vi "MGCC_MdlMgmt_Graphic.vi"() -> ()   [LabVIEW 2016]
doc: "-----------------------------------------------------------------------------------------------------------------------\nCopyright <2019> <The University of Tennessee at Knoxville and the University of Tennessee Research Foundation>\nThis software is released under BSD-3 \nhttps://opensource.org/licenses/BSD-3-Clause \nAdditional license options available at https://utrf.tennessee.edu/industry/sample-agreements/\n-----------------------------------------------------------------------------------------------------------------------\n\nThis VI is designed to initize the SHE215 model with graphic (2D double array).-----------------------------"
uses:
  <vilib>/imath/engines/lvmath2/RunTimeEngine/NodeEndStatement/NIMS_NodeEndStatement_Output.vi
  <instcachedir>/0/NIMS_NodeEndStatement_Output_53EC0D466D134D7ABD903AC30B43404B.lvgen/NIMS_NodeEndStatement_Output_53EC0D466D134D7ABD903AC30B43404B_010.vi
  <vilib>/imath/engines/lvmath2/RunTimeEngine/ErrorHandling/NIMS_Finalize Error.vi
panel:
  out "array":dbl[][](array[numeric])
  out "text":string
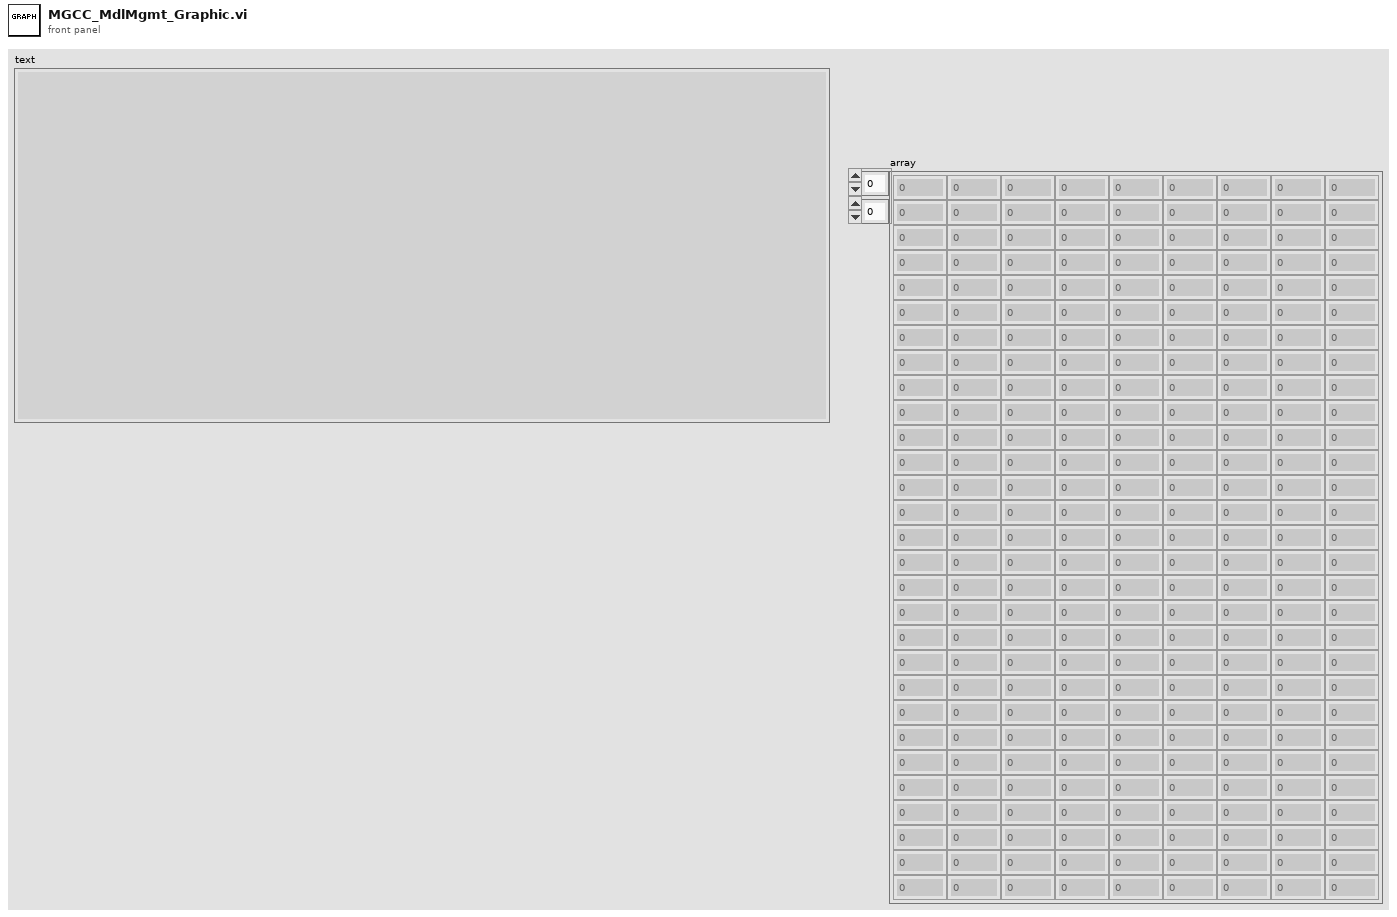
[diagram p1: front panel]
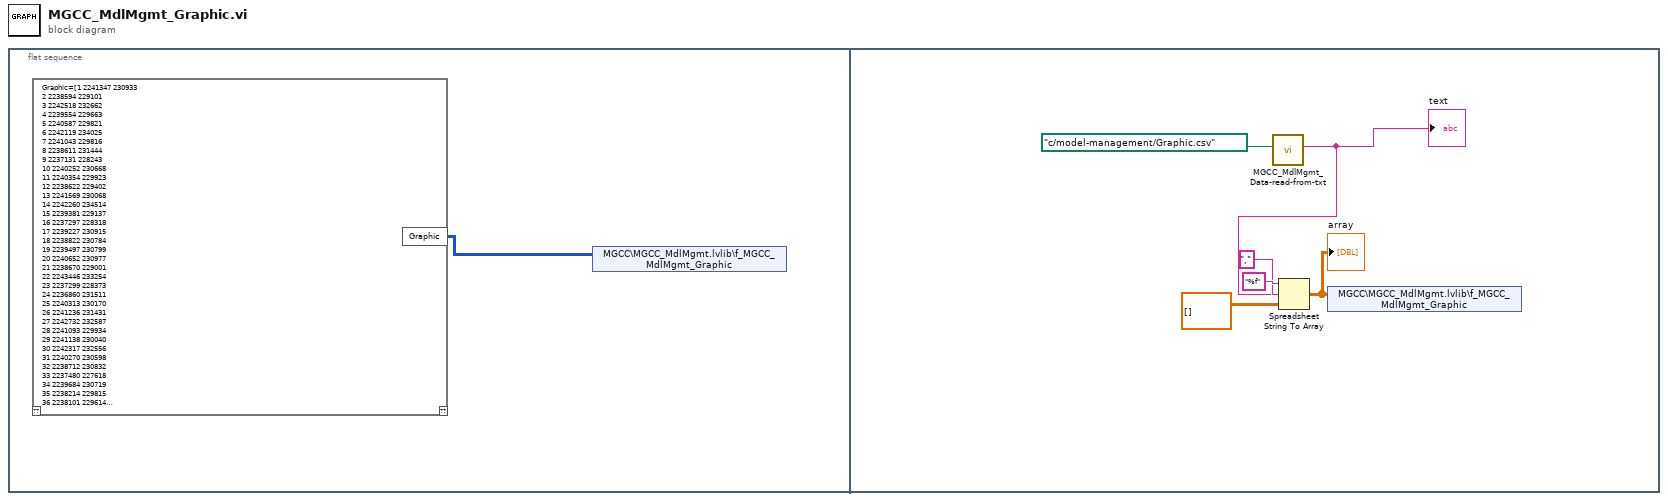
[diagram p0: block diagram]
diagram:
  n1 = flat-sequence {
    frame #0 {
      n2 = mathscript code="Graphic=[1\t2241347\t230933\n2\t2238594\t229101\n3\t2242518\t232662\n4\t2239554\t229663\n5\t2240587\t229821\n6\t2242119\t234025\n7\t2241043\t229816\n8\t2238611\t231444\n9\t2237131\t228243\n10\t2240252\t230668\n11\t2240354\t229923\n12\t2238622\t229402\n13\t2241569\t230068\n14\t2242260\t234514\n15\t2239381\t229137\n16\t2237297\t228318\n17\t2239227\t230915\n18\t2238822\t230784\n19\t2239497\t230799\n20\t2240652\t230977\n21\t2238670\t229001\n22\t2243446\t233254\n23\t2237299\t228373\n24\t2236860\t231511\n25\t2240313\t230170\n26\t2241236\t231431\n27\t2242732\t232587\n28\t2241093\t229934\n29\t2241138\t230040\n30\t2242317\t232556\n31\t2240270\t230598\n32\t2238712\t230832\n33\t2237480\t227618\n34\t2239684\t230719\n35\t2238214\t229815\n36\t2238101\t229614\n37\t2239201\t229854\n38\t2239291\t230583\n39\t2239052\t228410\n40\t2237867\t229724\n41\t2238322\t229509\n42\t2238145\t229033\n43\t2241409\t230629\n44\t2239661\t229599\n45\t2242631\t234355\n46\t2238950\t231034\n47\t2237485\t228516\n48\t2243165\t233311\n49\t2239827\t230147\n50\t2238730\t230867\n51\t2239618\t228552\n52\t2240805\t229721\n53\t2237071\t228122\n54\t2240553\t230476\n55\t2242445\t234436\n56\t2239862\t230630\n57\t2242511\t233856\n58\t2238251\t229036\n59\t2237800\t227534\n60\t2243409\t233119\n61\t2240015\t230483\n62\t2236935\t228092\n63\t2237312\t232477\n64\t2237562\t228888\n65\t2240884\t230680\n66\t2238941\t232437\n67\t2243265\t234127\n68\t2238371\t230913\n69\t2239407\t230840\n70\t2240819\t231106\n71\t2239293\t228944\n72\t2240694\t229147\n73\t2238608\t230876\n74\t2239967\t230467\n75\t2239254\t228857\n76\t2239884\t230123\n77\t2238139\t227705\n78\t2238429\t229814\n79\t2237539\t229577\n80\t2241020\t230274\n81\t2240648\t229500\n82\t2238544\t231292\n83\t2237163\t231970\n84\t2240407\t230787\n85\t2243126\t234150\n86\t2236331\t230503\n87\t2240695\t230810\n88\t2238013\t227700\n89\t2237806\t228632\n90\t2238369\t229205\n91\t2237392\t229065\n92\t2241605\t232088\n93\t2240971\t230678\n94\t2238496\t229227\n95\t2242252\t233968\n96\t2241024\t229627\n97\t2237160\t228190\n98\t2239057\t230683\n99\t2241692\t231790\n100\t2238315\t229898\n101\t2241513\t230126\n102\t2240441\t230483\n103\t2242556\t232451\n104\t2238193\t229569\n105\t2237909\t228485\n106\t2237588\t229745\n107\t2240416\t230399\n108\t2238691\t229455\n109\t2239672\t230218\n110\t2236545\t230430\n111\t2238502\t231201\n112\t2241109\t229619\n113\t2237475\t228378\n114\t2238404\t230985\n115\t2239460\t229314\n116\t2237463\t229313\n117\t2240662\t230430\n118\t2236585\t227775\n119\t2241301\t231156\n120\t2237758\t228734\n121\t2239041\t230995\n122\t2236537\t230356\n123\t2236982\t227856\n124\t2239904\t230328\n125\t2237593\t229764\n126\t2238822\t231087\n127\t2243437\t233385\n128\t2240694\t230934\n129\t2238929\t231349\n130\t2241383\t230757\n131\t2240228\t229979\n132\t2239104\t228525\n133\t2243389\t233847\n134\t2236970\t228044\n135\t2240458\t229249\n136\t2237802\t227555\n137\t2238822\t229476\n138\t2237406\t228378\n139\t2241100\t229599\n140\t2239788\t228942\n141\t2242888\t234252\n142\t2240379\t230317\n143\t2237539\t228300\n144\t2239271\t229185\n145\t2236506\t230371\n146\t2236757\t227878\n147\t2238506\t229643\n148\t2240011\t230580\n149\t2240999\t229712\n150\t2243272\t234087\n151\t2237850\t227910\n152\t2237128\t231945\n153\t2242901\t232717\n154\t2236312\t230462\n155\t2240039\t229436\n156\t2237498\t229438\n157\t2241100\t231247\n158\t2240856\t230345\n159\t2239673\t228677\n160\t2238499\t229306\n161\t2239171\t228674\n162\t2241801\t231876\n163\t2241419\t230644\n164\t2237651\t228167\n165\t2241934\t232688\n166\t2239653\t229002\n167\t2241022\t231263\n168\t2241891\t234123\n169\t2243556\t233778\n170\t2237387\t228440\n171\t2236902\t227959\n172\t2236849\t231114\n173\t2238907\t232116\n174\t2239695\t229844\n175\t2238768\t229516\n176\t2236864\t227960\n177\t2242040\t232053\n178\t2237639\t229831\n179\t2240087\t230455\n180\t2241449\t230437\n181\t2240583\t229195\n182\t2242723\t233763\n183\t2240756\t230390\n184\t2240736\t230166\n185\t2242528\t234106\n186\t2243117\t232884\n187\t2243400\t233101\n188\t2239885\t229503\n189\t2243413\t234038\n190\t2240702\t230089\n191\t2236702\t227897\n192\t2239726\t228800\n193\t2239178\t229884\n194\t2238296\t229149\n195\t2239531\t229475\n196\t2239198\t229219\n197\t2239865\t230367\n198\t2237976\t227619\n199\t2240693\t229602\n200\t2236666\t230842\n201\t2238390\t229145\n202\t2240924\t229671\n203\t2237641\t227582\n204\t2237660\t228651\n205\t2238243\t228980\n206\t2238114\t229733\n207\t2242322\t232271\n208\t2240781\t230727\n209\t2243537\t233574\n210\t2240334\t229309\n211\t2238986\t229686\n212\t2238761\t231780\n213\t2240183\t229374\n214\t2242378\t233912\n215\t2239549\t229047\n216\t2239087\t230347\n217\t2242186\t232811\n218\t2238887\t231246\n219\t2241691\t230110\n220\t2240294\t229632\n221\t2239509\t230092\n222\t2239440\t229669\n223\t2241054\t229771\n224\t2238545\t231548\n225\t2242078\t234593\n226\t2238724\t229208\n227\t2237228\t228463\n228\t2240255\t230214\n229\t2241437\t231590\n230\t2242547\t232627\n231\t2241155\t230014\n232\t2239397\t230006\n233\t2238911\t228206\n234\t2238010\t229196\n235\t2241502\t230580\n236\t2240443\t230989\n237\t2243151\t233303\n238\t2239564\t228419\n239\t2240723\t229671\n240\t2240344\t229751\n241\t2237435\t232775\n242\t2238264\t230581\n243\t2239769\t230012\n244\t2240915\t229052\n245\t2240032\t230061\n246\t2241110\t230236\n247\t2238051\t228617\n248\t2238185\t229276\n249\t2237391\t228968\n250\t2241555\t232081\n251\t2240905\t230495\n252\t2241659\t232094\n253\t2238349\t229902\n254\t2237903\t228844\n255\t2241512\t229827\n256\t2237789\t228353\n257\t2238461\t231108\n258\t2241212\t229624\n259\t2237244\t229365\n260\t2241257\t231320\n261\t2236629\t230311\n262\t2238878\t231372\n263\t2239857\t230607\n264\t2243365\t233854\n265\t2237763\t227649\n266\t2238961\t229402\n267\t2238914\t229295\n268\t2240666\t230006\n269\t2241110\t229449\n270\t2242759\t234308\n271\t2239352\t229286\n272\t2236352\t230443\n273\t2240050\t230669\n274\t2236424\t227529\n275\t2243409\t234029\n276\t2237916\t227970\n277\t2239956\t229205\n278\t2241154\t231231\n279\t2237753\t228036\n280\t2241930\t232705\n281\t2241330\t231165\n282\t2238825\t232060\n283\t2241540\t230615\n284\t2238651\t229348\n285\t2240145\t230450\n286\t2240554\t229038\n287\t2241085\t230323\n288\t2242693\t233630\n289\t2242995\t232992\n290\t2243545\t234005\n291\t2239287\t229951\n292\t2239095\t229287\n293\t2236837\t227611\n294\t2238251\t228920\n295\t2241049\t230793\n296\t2240831\t229458\n297\t2238883\t230108\n298\t2241929\t233062\n299\t2241655\t230313];"() -> ("Graphic"=w1:i32[][])  [unwired: 1 in, 1 out]
      n3 = shared-variable "MGCC\\MGCC_MdlMgmt.lvlib\\f_MGCC_MdlMgmt_Graphic"(w1) -> ()  [unwired: 1 in, 1 out]
    }
    frame #1 {
      n4 = call "MGCC_MdlMgmt_Data-read-from-txt.vi"("file path (use dialog)"=path "c:/model-management/Graphic.csv") -> ("text"=w15:string)  [unwired: 10 in]
      "text" <- w15
      n5 = Spreadsheet String To Array(delimiter (Tab)=",", format string="%f", spreadsheet string=w15, array type (2D Dbl)=dbl[][] []) -> (array=w16:dbl[][])
      "array" <- w16
      n6 = shared-variable "MGCC\\MGCC_MdlMgmt.lvlib\\f_MGCC_MdlMgmt_Graphic"(w16) -> ()  [unwired: 1 in, 1 out]
    }
  }
